vi "_io_query.vi"(4 "Simulation read buffer (\"Simulation\")":string="Simulation", 6 "Block Logging (F)":bool, 7 "Allow Assure End with LF":bool=TRUE, 8 "error in":errorcluster caption="error in (no error)", 9 "Max bytes to read (2048)":u32=2048, 10 "Write buffer":string, 11 "VISA resource name":refnum<visa-resource-name>) -> (0 "error out":errorcluster, 1 "Read bytes count":u32, 2 "Read buffer":string, 3 "VISA resource name out":refnum<visa-resource-name>)   [LabVIEW 2022 SP3, in "hmp4000_rsidr_core.lvlib"]
uses:
  hmp4000_rsidr_core.lvlib
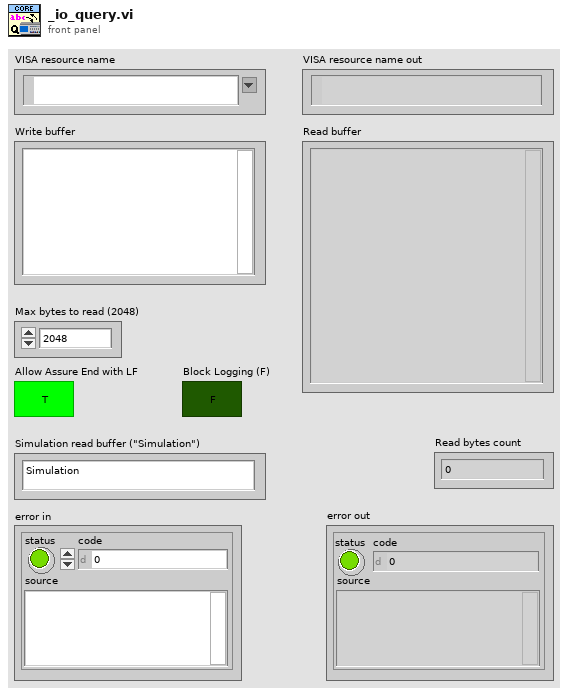
[diagram p1: front panel]
types:
  T1 = typedef "hmp4000_rsidr_core.lvlib/type_Session_Data.ctl" = cluster{"IDN string":string, "Instrument FW":string, "Instr type":string, "Instr type for err. msg.":string, "Installed Options":string[], "Ignore Error Messages":string, "Logging params":variant, "OPC Timeout":i32, "VISA Timeout":i32, "STB Poll VISA Timeout":i32, "Additional Flags":i32, "Wait Before Read":i32, "Wait Before Write":i32, "Option String Flags":i32, "IO Segment Size":i64, "VISA Access Mode":T2, "Interface Type":T3, "OPC Wait Mode":T4, "Bin Float Number  Format":T5, "Bin Integer Number Format":T6, "Simulate":bool, "VXIcapable":bool, "Duplicate Session":bool, "Add LF to Write":bool, "Logging":bool, "Fast Sweep":bool, "Query Instrument Status":bool, "Check Range":bool, "Check Options":bool}
  T2 = typedef "hmp4000_rsidr_core.lvlib/type_VisaAccessMode.ctl" = u16
  T3 = typedef "hmp4000_rsidr_core.lvlib/type_InterfaceType.ctl" = enum16{"Unknown", "GPIB", "VXI", "GPIB_VXI", "ASRL", "PXI", "TCPIP", "USB", "SOCKET"}
  T4 = typedef "hmp4000_rsidr_core.lvlib/type_OPC_Wait_Mode.ctl" = enum16{"STBpolling", "STBpollingSlow", "STBpollingSuperSlow", "ServiceRequest", "OPCquery"}
  T5 = typedef "hmp4000_rsidr_core.lvlib/type_Binary_Float_Number_Format.ctl" = enum16{"Float_4_Bytes_Swapped", "Float_4_Bytes", "Double_8_Bytes_Swapped", "Double_8_Bytes"}
  T6 = typedef "hmp4000_rsidr_core.lvlib/type_Binary_Integer_Number_Format.ctl" = enum16{"Int32_4_Bytes_Swapped", "Int32_4 Bytes", "Int16_2_Bytes_Swapped", "Int16_2_Bytes"}
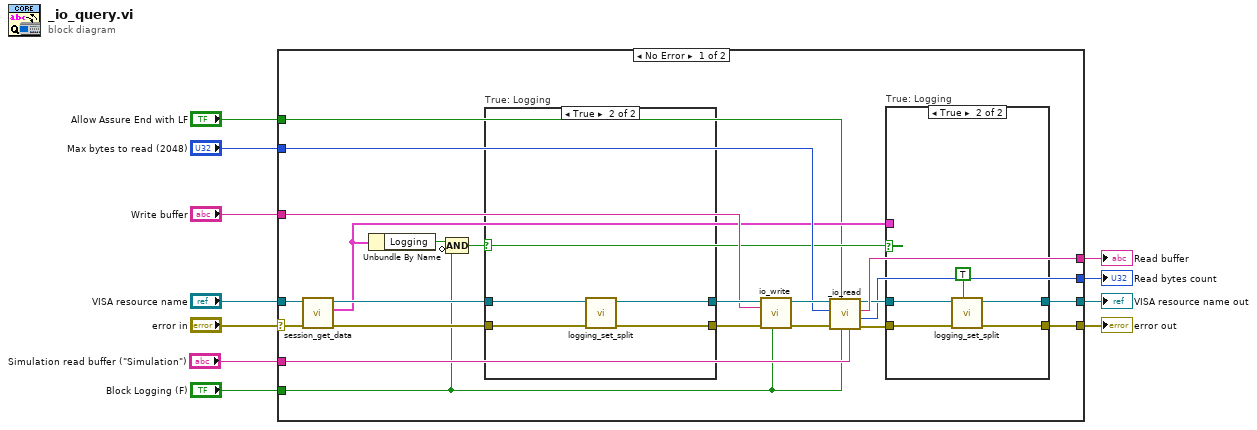
[diagram p0: block diagram]
diagram:
  n1 = case shown="No Error" "error in" {
    selector: "error in" -> [w26 w48]
    tunnel: [w21 w47] -> w7
    tunnel: [w22 w48] -> w3
    tunnel: "Write buffer" -> [w27 _]
    tunnel: "VISA resource name" -> [w25 w47]
    tunnel: "Block Logging (F)" -> [w13 _]
    tunnel: "Max bytes to read (2048)" -> [w28 _]
    tunnel: "Simulation read buffer (\"Simulation\")" -> [w17 _]
    tunnel: [w29 _] -> w6
    tunnel: [w16 _] -> w2
    tunnel: "Allow Assure End with LF" -> [w12 _]
    frame No Error {
      n2 = call "session_get_data.vi"("error in"=w26, "VISA resource name"=w25) -> ("error out"=w24:errorcluster, "Session User Data out"=w18:T1, "VISA resource name out"=w23:refnum<visa-resource-name>)  [unwired: 6 in, 1 out]
      n3 = Unbundle By Name(w18) -> ("Logging"=w15:bool)
      n4 = Compound Arithmetic op=AND(w15, invert w13) -> (w14:bool)
      n5 = case "True: Logging" shown="True" w14 {
        tunnel: w24 -> [w42 w46]
        tunnel: w23 -> [w41 w45]
        tunnel: [w42 w43] -> w30
        tunnel: [w41 w44] -> w31
        frame False {
        }
        frame True {
          n6 = call "logging_set_split.vi"("error in"=w46, "VISA resource name"=w45) -> ("error out"=w43:errorcluster, "VISA resource name out"=w44:refnum<visa-resource-name>)  [unwired: 8 in]
        }
      }
      n7 = call "io_write.vi"("Block Logging (F)"=w13, "error in"=w30, "write buffer"=w27, "VISA resource name"=w31) -> ("error out"=w32:errorcluster, "VISA resource name out"=w33:refnum<visa-resource-name>)  [unwired: 6 in]
      n8 = call "_io_read.vi"("Simulation read buffer (\"Simulation\")"=w17, "Block Logging (F)"=w13, "Allow Assure End with LF"=w12, "error in"=w32, "Max bytes to read (2048)"=w28, "VISA resource name"=w33) -> ("error out"=w20:errorcluster, "Read bytes count"=w16:u32, "Read buffer"=w29:string, "VISA resource name out"=w19:refnum<visa-resource-name>)  [unwired: 2 in]
      n9 = case "True: Logging" shown="True" w14 {
        tunnel: w20 -> [w35 w40]
        tunnel: [w35 w38] -> w22
        tunnel: w19 -> [w34 w39]
        tunnel: [w34 w37] -> w21
        tunnel: w18 -> [_ _]
        frame False {
        }
        frame True {
          n10 = call "logging_set_split.vi"("Evaluate section error (F)"=TRUE, "error in"=w40, "VISA resource name"=w39) -> ("error out"=w38:errorcluster, "VISA resource name out"=w37:refnum<visa-resource-name>)  [unwired: 7 in]
        }
      }
    }
    frame Error {
    }
  }
  "VISA resource name out" <- w7
  "error out" <- w3
  "Read buffer" <- w6
  "Read bytes count" <- w2
